vi "PDWV Partial density of Water Vapor (kg to m3).vi"(1 "Tceg":dbl[unit], 2 "RH":dbl) -> (0 "PDWV":dbl[unit])   [LabVIEW 2018]
panel:
  out "R 2":dbl[unit]
  out "s^-2 m^2 kg K^-1 mol^-1":dbl[unit]
  out "R":dbl[unit]
  out "M-W 3":dbl[unit]=0.018
  out "PDWV\nPartial density of Water Vapor\nPDWV=(PPWV*M_W)/(R*Tk)":dbl[unit](knob) scale=0.0..0.6
  out "Temprature Of Input Air\nKelvin Degree":dbl[unit](slide) scale=273.0..373.0
  out "Tk":dbl[unit]
  out "Temprature Of Input Air\nCentigrade Degree":dbl[unit](slide) scale=0.0..100.0
  out "Humidity of Input Air":dbl(knob) scale=0.0..100.0
  out "M-W 2":dbl[unit]=0.018
  out "M-W":dbl[unit]=0.018
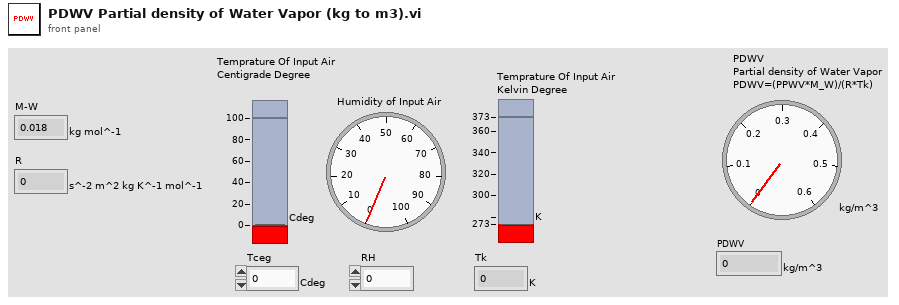
[diagram p1: front panel]
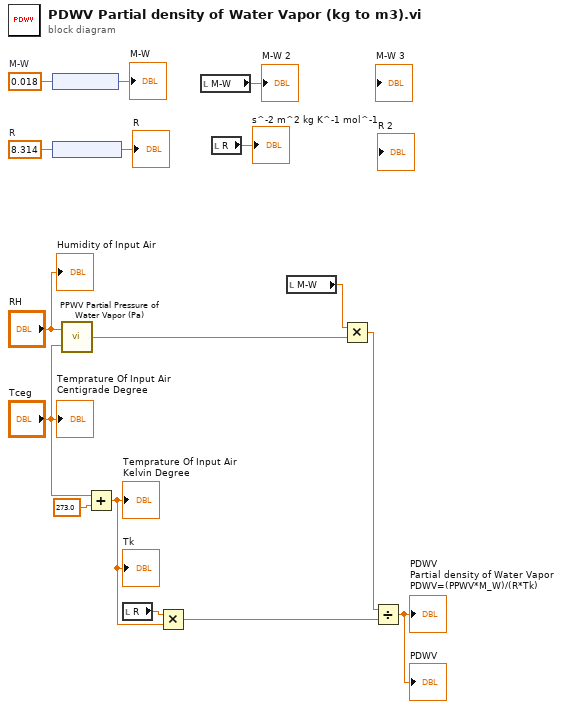
[diagram p0: block diagram]
diagram:
  w10 = 8.314  # R
  w15 = 0.018  # M-W
  n1 = node(w15) -> (→"M-W":dbl[unit])
  n2 = node ("Convert Unit")(w10) -> (→"R":dbl[unit])
  n3 = call "PPWV Partial Pressure of Water Vapor (Pa).vi"("Tceg"="Tceg", "RH"="RH") -> ("PPWV"=w3:dbl[unit])
  n4 = Add(x="Tceg", y=dbl[unit] 273.0) -> (x+y=w4:dbl[unit])
  "Tk" <- w4
  "Temprature Of Input Air\nKelvin Degree" <- w4
  n5 = local read "R"() -> (w5:dbl[unit])
  n6 = Multiply(x=w5, y=w4) -> (x*y=w8:dbl[unit])
  n7 = local read "M-W"() -> (→"M-W 2":dbl[unit])
  n8 = local read "R"() -> (→"s^-2 m^2 kg K^-1 mol^-1":dbl[unit])
  n9 = local read "M-W"() -> (w12:dbl[unit])
  n10 = Multiply(x=w12, y=w3) -> (x*y=w11:dbl[unit])
  n11 = Divide(x=w11, y=w8) -> (x/y=→"PDWV\nPartial density of Water Vapor\nPDWV=(PPWV*M_W)/(R*Tk)" →"PDWV":dbl[unit])
  "Humidity of Input Air" <- "RH"
  "Temprature Of Input Air\nCentigrade Degree" <- "Tceg"
